vi "Module Type.vi"(11 "OtherModule in":refnum<class "OtherModule.lvclass">) -> (2 "Module Type":string)   [LabVIEW 2020, in "VolatusScratch.lvlib" / "OtherModule.lvclass"]
uses:
  OtherModule.lvclass
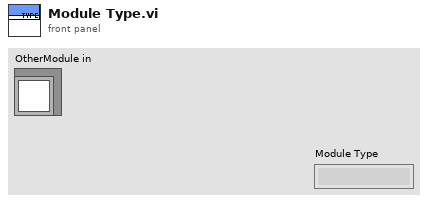
[diagram p1: front panel]
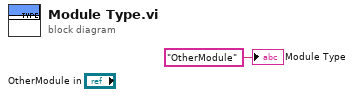
[diagram p0: block diagram]
diagram:
  "Module Type" <- "OtherModule" ("Module Type")
